vi "Drive Control (SubVI).vi"(7 "H Tank Disabled":bool, 8 "Buttons":bool[](array[boolean]), 9 "Joystick Axis":dbl[](array[numeric]), 10 "PID gains Slow":T1={"proportional gain (Kc)"=0.7500000000000001, "integral time (Ti, min)"=0.004, "derivative time (Td, min)"=0.0} {"derivative time (Td, min)" format="%.3f"; "integral time (Ti, min)" format="%.3f"; "proportional gain (Kc)" format="%.3f"}, 11 "PID gains Fast":T1={"proportional gain (Kc)"=0.7500000000000001, "integral time (Ti, min)"=0.001, "derivative time (Td, min)"=0.0} {"derivative time (Td, min)" format="%.3f"; "integral time (Ti, min)" format="%.3f"; "proportional gain (Kc)" format="%.3f"}) -> ()   [LabVIEW 2014]
uses:
  <vilib>/Rock Robotics/WPI/Solenoid/WPI_SolenoidValue.ctl
  <vilib>/Rock Robotics/WPI/RobotDrive/WPI_RobotDriveGetSetRefNum.vi
  <vilib>/addons/control/pid/pid.llb/PID Control Input Filter (DBL).vi
  <vilib>/Rock Robotics/WPI/Solenoid/WPI_SolenoidSetEnum.vi
  <vilib>/addons/control/pid/pid.llb/PID (DBL).vi
  <vilib>/Rock Robotics/Network Tables/SD Write Numeric Array.vi
  <vilib>/addons/control/pid/NI_PID_pid.lvlib
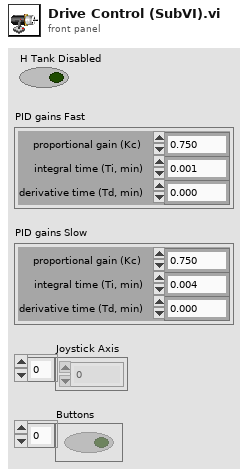
[diagram p1: front panel]
types:
  T1 = cluster{"proportional gain (Kc)":dbl, "integral time (Ti, min)":dbl, "derivative time (Td, min)":dbl}
  T2 = typedef "WPI_SolenoidValue.ctl" = enum16{"Off", "On", "Forward", "Reverse"}
  T3 = typedef "WPI_RobotDriveDevRef.ctl" = cluster{"DevStatus":errorcluster, "Motors[]":T4[], "Square Inputs":bool, "Max Output":dbl}
  T4 = typedef "WPI_MotorControlDeviceRef.ctl" = cluster{"DeviceStatus":errorcluster, "Type":T5, "PWM":cluster{"Controller":T6, "PWM Channel":T7, "DeadBand":T8}, "CAN":cluster{"Device Number":u8, "Control Mode":T9, "Semaphore":T10, "Max Vout":dbl, "TalonSRX Control Mode":T11}, "Invert":bool, "TransformRef":T12, "InvTransformRef":T12}
  T5 = typedef "WPI_MotorControlType.ctl" = enum16{"PWM", "CAN", "CANTalonSRX"}
  T6 = typedef "FPGA_TypedefDigitalModule.ctl" = enum16{"Controller 1"}
  T7 = typedef "FPGA_DIOPWMChannel.ctl" = enum8{"PWM 0", "PWM 1", "PWM 2", "PWM 3", "PWM 4", "PWM 5", "PWM 6", "PWM 7", "PWM 8", "PWM 9", "PWM MXP 0", "PWM MXP 1", "PWM MXP 2", "PWM MXP 3", "PWM MXP 4", "PWM MXP 5", "PWM MXP 6", "PWM MXP 7", "PWM MXP 8", "PWM MXP 9", "Invalid"}
  T8 = typedef "WPI_PWMDeadband.ctl" = cluster{"Name":string, "maxPositivePwm":i32, "minPositivePwm":i32, "centerPwm":i32, "maxNegativePwm":i32, "minNegativePwm":i32, "angularRange":u16}
  T9 = typedef "WPI_CANJaguar_ControlMode.ctl" = enum8{"Percent VBus", "Current", "Speed", "Position", "Voltage"}
  T10 = typedef "Semaphore RefNum" = refnum<k1>
  T11 = typedef "WPI_CANTalonSRX_APIControlMode.ctl" = enum8{"Percent VBus", "Speed", "Position", "Slave", "Unchanged / Invalid"}
  T12 = typedef "WPI_PWMTransform_ConPane.ctl" = refnum<vi>
  T13 = typedef "WPI_SolenoidDevRef.ctl" = cluster{"DevStatus":errorcluster, "Pneumatics Control Module":u8, "Forward Solenoid Channel":T14, "Reverse Solenoid Channel":T14}
  T14 = typedef "WPI_SolenoidChannel.ctl" = enum8{"Solenoid 0", "Solenoid 1", "Solenoid 2", "Solenoid 3", "Solenoid 4", "Solenoid 5", "Solenoid 6", "Solenoid 7", "Invalid"}
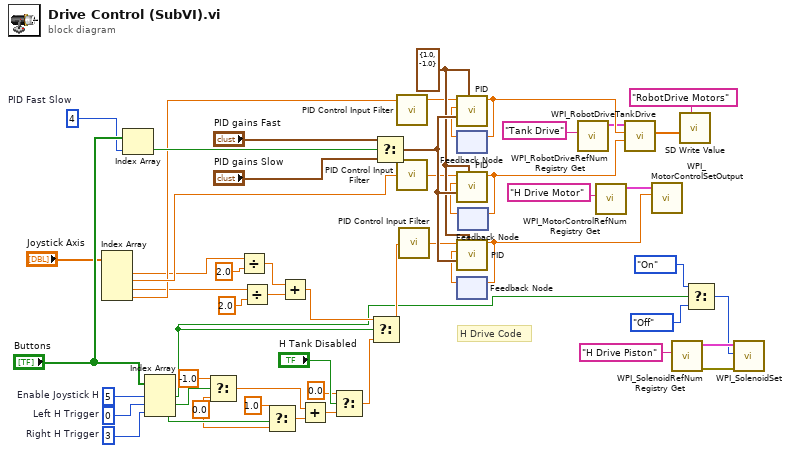
[diagram p0: block diagram]
diagram:
  w52 = 4  # PID Fast Slow
  w51 = 3  # Right H Trigger
  w48 = 0  # Left H Trigger
  w47 = 5  # Enable Joystick H
  w41 = cluster{"output high":dbl, "output low":dbl} {"output high"=1.0, "output low"=-1.0} ("output range")
  w22 = 0.0 ("t")
  # "H Drive Code"
  n1 = Index Array(array="Joystick Axis") -> (element #1=w12:dbl, element #2=w46:dbl, element #3=w13:dbl, element #4=w38:dbl)  [unwired: 4 in]
  n2 = Index Array ("H Drive Triggers")(array="Buttons", index=w52) -> (element=w54:bool)
  n3 = Index Array ("H Drive Triggers")(array="Buttons", index #1=w47, index #2=w48, index #3=w51) -> (element #1=w1:bool, element #2=w50:bool, element #3=w49:bool)
  n4 = Select(t=-1.0, s=w50, f=w22) -> (s? t:f=w21:dbl)
  n5 = Divide(x=w12, y=2.0) -> (x/y=w16:dbl)
  n6 = Divide(x=w13, y=2.0) -> (x/y=w14:dbl)
  n7 = Select(t=1.0, s=w49, f=w22) -> (s? t:f=w20:dbl)
  n8 = Add(x=w16, y=w14) -> (x+y=w42:dbl)
  n9 = Add(x=w21, y=w20) -> (x+y=w19:dbl)
  n10 = Select(t=0.0 ("f"), s="H Tank Disabled", f=w19) -> (s? t:f=w18:dbl)
  n11 = Select(t=w42, s=w1, f=w18) -> (s? t:f=w44:dbl)
  n12 = Select(t="PID gains Fast", s=w54, f="PID gains Slow") -> (s? t:f=w43:T1)
  n13 = call-poly <vilib>:"PID Control Input Filter.vi"("input"=w38) -> ("output"=w32:dbl)  [unwired: 4 in]
  n14 = call-poly <vilib>:"PID Control Input Filter.vi"("input"=w46) -> ("output"=w31:dbl)  [unwired: 4 in]
  n15 = call-poly <vilib>:"PID Control Input Filter.vi"("input"=w44) -> ("output"=w39:dbl)  [unwired: 4 in]
  n16 = feedback #1() -> (w33:dbl)  [unwired: 1 in]
  n17 = call-poly <vilib>:"PID.vi"("output range"=w41, "PID gains"=w43, "process variable"=w33, "setpoint"=w32) -> ("output"=w34:dbl)  [unwired: 6 in, 1 out]
  n18 = feedback-in #1(w34) -> ()
  n19 = feedback #2() -> (w40:dbl)  [unwired: 1 in]
  n20 = call-poly <vilib>:"PID.vi"("output range"=w41, "PID gains"=w43, "process variable"=w40, "setpoint"=w39) -> ("output"=w5:dbl)  [unwired: 6 in, 1 out]
  n21 = feedback-in #2(w5) -> ()
  n22 = feedback #3() -> (w30:dbl)  [unwired: 1 in]
  n23 = call-poly <vilib>:"PID.vi"("output range"=w41, "PID gains"=w43, "process variable"=w30, "setpoint"=w31) -> ("output"=w35:dbl)  [unwired: 6 in, 1 out]
  n24 = feedback-in #3(w35) -> ()
  n25 = call <vilib>:"WPI_RobotDriveRefNum Registry Get.vi"("refnum name"="Tank Drive") -> ("RobotDriveDevRef"=w29:T3)  [unwired: 1 in, 9 out]
  n26 = call <vilib>:"WPI_MotorControlRefNum Registry Get.vi"("refnum name"="H Drive Motor") -> ("MotorControlDevRef"=w27:T4)  [unwired: 9 in, 1 out]
  n27 = call <vilib>:"WPI_RobotDriveTankDrive.vi"("Right axis value"=w35, "Left axis value"=w34, "RobotDriveDevRef"=w29) -> ("Motor Values"=w11:dbl[])  [unwired: 6 in, 2 out]
  n28 = call <vilib>:"WPI_MotorControlSetOutput.vi"("Output"=w5, "MotorControlDevRef"=w27) -> ()  [unwired: 7 in, 3 out]
  n29 = call <vilib>:"WPI_SolenoidRefNum Registry Get.vi"("refnum name"="H Drive Piston") -> ("error out"=w7:errorcluster, "SolenoidDevRef"=w6:T13)  [unwired: 9 in]
  n30 = call-poly <vilib>:"SD Write Value.vi"("Numeric Array"=w11, "Name"="RobotDrive Motors") -> ()  [unwired: 8 in, 2 out]
  n31 = Select(t=WPI_SolenoidValue."On" ("Value"), s=w1, f=WPI_SolenoidValue."Off" ("Value")) -> (s? t:f=w2:T2)
  n32 = call-poly <vilib>:"WPI_SolenoidSet.vi"("error in (no error)"=w7, "Value"=w2, "SolenoidDevRef"=w6) -> ()  [unwired: 7 in, 2 out]
